vi "VLC - Play Stream&Snapshot.vi"(5 "Media Source":string="rtsp://user:password@*.*.*.*/axis-media/media.amp?videocodec=h264", 7 "Script":string, 11 "error in (no error)":errorcluster) -> (15 "error out":errorcluster)   [LabVIEW 2012]
uses:
  <vilib>/Utility/sysdir.llb/System Directory Type.ctl
  System.Windows.Forms
panel:
  in  "PictureBox":refnum<k24>(container)
  in  "Snap":bool
  # "http://www.videolan.org/developers/vlc/doc/doxygen/html/modules.html"
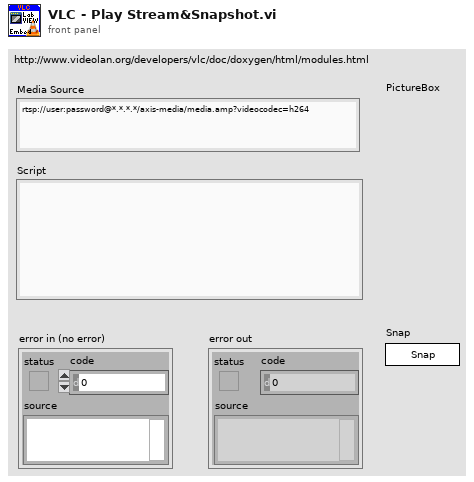
[diagram p1: front panel]
types:
  T1 = typedef "System Directory Type.ctl" = i32
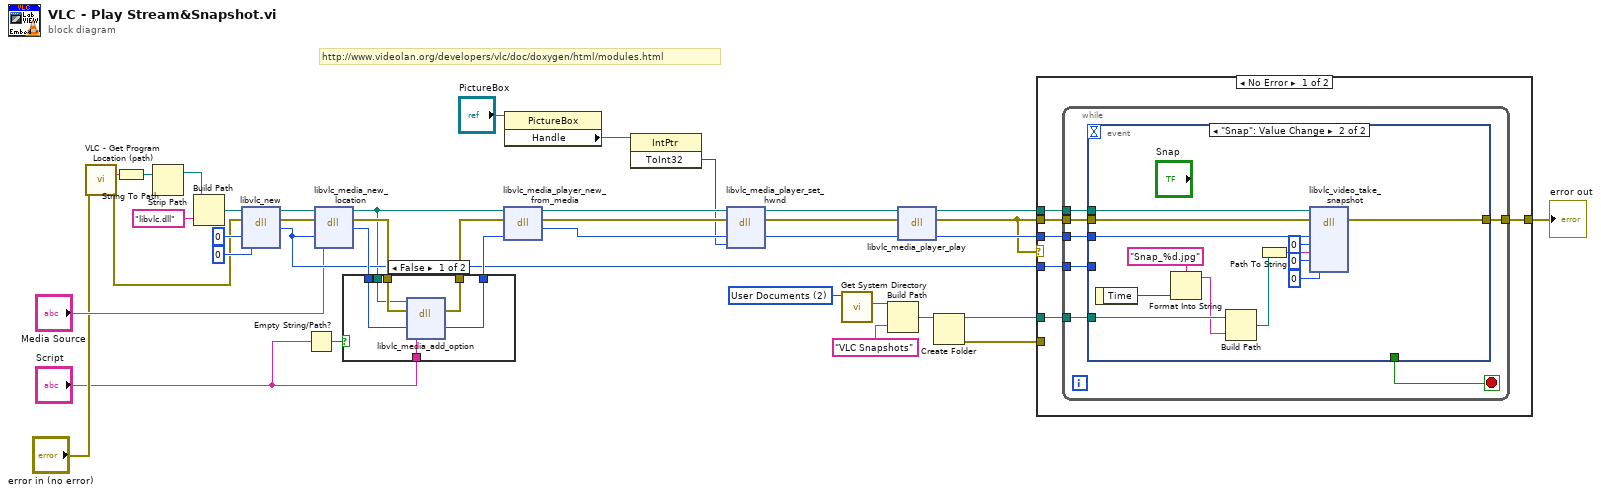
[diagram p0: block diagram]
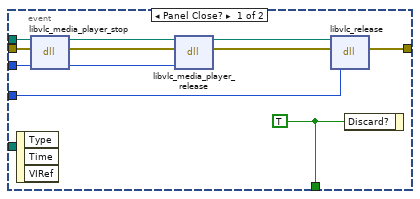
[diagram p2: hidden frame]
diagram:
  w6 = T1 2 items=["User Home"=0, "User Desktop"=1, "User Documents"=2, "User Application Data"=3, "User Preferences"=4, "User Temporary"=5, "Public Documents"=6, "Public Application Data"=7, "Public Preferences"=8, "Public Cache"=13, "System Core Libraries"=9, "System Installed Libraries"=10, "Application Files"=11, "Boot Volume Root"=12] ("system directory type")
  # "http://www.videolan.org/developers/vlc/doc/doxygen/html/modules.html"
  n1 = call "VLC - Get Program Location (path).vi"("error in (no error)"="error in (no error)") -> ("VLC path"=w22:string, "error out"=w15:errorcluster)  [unwired: 13 in]
  n2 = String To Path(string=w22) -> (path=w21:path)
  n3 = Strip Path(path=w21) -> (stripped path=w20:path)  [unwired: 1 out]
  n4 = Build Path(base path=w20, name or relative path="libvlc.dll") -> (appended path=w18:path)
  n5 = dll-call lib="C:/Program Files (x86)/VideoLAN/VLC/libvlc.dll" fn="libvlc_new"(path in=w18, error in=w15, "argc"=i16 0, "argv"=u8 0) -> (path out=w26:path, error out=w29:errorcluster, "return type"=w35:i32)  [unwired: 3 in]
  n6 = Empty String/Path?(string/path="Script") -> (empty?=w13:bool)
  n7 = dll-call lib="C:/Program Files (x86)/VideoLAN/VLC/libvlc.dll" fn="libvlc_media_new_location"(path in=w26, error in=w29, "p_instance"=w35, "path"="Media Source") -> (path out=w10:path, error out=w36:errorcluster, "return type"=w37:i32)  [unwired: 3 in]
  n8 = case shown="False" w13 {
    tunnel: w36 -> [w45 w47]
    tunnel: w37 -> [w44 w46]
    tunnel: [w43 w46] -> w38
    tunnel: [w42 w47] -> w39
    tunnel: "Script" -> [w41 _]
    tunnel: w10 -> [w40 _]
    frame False {
      n9 = dll-call lib="C:/Program Files (x86)/VideoLAN/VLC/libvlc.dll" fn="libvlc_media_add_option"(path in=w40, error in=w45, "p_md"=w44, "ppsz_options"=w41) -> (error out=w42:errorcluster, "p_md"=w43:i32)  [unwired: 3 in, 1 out]
    }
    frame True {
    }
  }
  n10 = dll-call lib="C:/Program Files (x86)/VideoLAN/VLC/libvlc.dll" fn="libvlc_media_player_new_from_media"(path in=w10, error in=w39, "p_md"=w38) -> (path out=w25:path, error out=w32:errorcluster, "return type"=w30:i32)  [unwired: 2 in]
  n11 = property class="PictureBox"(reference="PictureBox") -> ("Handle"=w8:refnum<k24>)  [unwired: 1 in, 2 out]
  n12 = invoke class="IntPtr" method="ToInt32"(reference=w8) -> ("ToInt32"=w7:i32)  [unwired: 2 in, 2 out]
  n13 = dll-call lib="C:/Program Files (x86)/VideoLAN/VLC/libvlc.dll" fn="libvlc_media_player_set_hwnd"(path in=w25, error in=w32, "p_mi"=w30, "drawable"=w7) -> (path out=w24:path, error out=w33:errorcluster, "p_mi"=w31:i32)  [unwired: 3 in]
  n14 = call <vilib>:"Get System Directory.vi"("system directory type"=w6) -> ("system directory"=w5:path)  [unwired: 10 in]
  n15 = Build Path(base path=w5, name or relative path="VLC Snapshots") -> (appended path=w3:path)
  n16 = dll-call lib="C:/Program Files (x86)/VideoLAN/VLC/libvlc.dll" fn="libvlc_media_player_play"(path in=w24, error in=w33, "p_mi"=w31) -> (path out=w23:path, error out=w11:errorcluster, "p_mi"=w34:i32)  [unwired: 2 in]
  n17 = Create Folder(path (use dialog)=w3) -> (created path=w2:path, error out=w1:errorcluster)  [unwired: 2 in, 1 out]
  n18 = case shown="No Error" w11 {
    tunnel: w35 -> [w53 _]
    tunnel: w34 -> [w52 _]
    tunnel: w11 -> [w51 w85]
    tunnel: w23 -> [w50 _]
    tunnel: [w49 w85] -> w12
    tunnel: w2 -> [w48 _]
    tunnel: w1 -> [_ _]
    frame No Error {
      n19 = while {
        tunnel: w53 -> [w60]
        tunnel: w52 -> [w59]
        tunnel: w51 -> [w58]
        tunnel: w50 -> [w57]
        tunnel: [w56] -> w49
        tunnel: w48 -> [w54]
        stop <- w55 stop-if-true
        n20 = event shown="[1] \"Snap\": Value Change" {
          selector: _ -> [_ _]
          dyn-events: _ -> [_ _]
          timeout: _ -> [_ _]
          tunnel: w58 -> [w71 w79]
          tunnel: w59 -> [w70 w77]
          tunnel: w60 -> [w66 _]
          tunnel: w57 -> [w65 w80]
          tunnel: [w62 w78] -> w56
          tunnel: [w61 _] -> w55
          tunnel: w54 -> [_ w74]
          event Panel Close? {
            w61 = TRUE ("Discard?")
            n21 = event-data() -> ()  [unwired: 1 in, 3 out]
            n22 = dll-call lib="C:/Program Files (x86)/VideoLAN/VLC/libvlc.dll" fn="libvlc_media_player_stop"(path in=w65, error in=w71, "p_mi"=w70) -> (path out=w64:path, error out=w69:errorcluster, "p_mi"=w68:i32)  [unwired: 2 in]
            n23 = dll-call lib="C:/Program Files (x86)/VideoLAN/VLC/libvlc.dll" fn="libvlc_media_player_release"(path in=w64, error in=w69, "p_mi"=w68) -> (path out=w63:path, error out=w67:errorcluster)  [unwired: 3 in]
            n24 = dll-call lib="C:/Program Files (x86)/VideoLAN/VLC/libvlc.dll" fn="libvlc_release"(path in=w63, error in=w67, "p_instnace"=w66) -> (error out=w62:errorcluster)  [unwired: 3 in, 1 out]
            n25 = event-data("Discard?"=w61) -> ()  [unwired: 1 in, 1 out]
          }
          event "Snap": Value Change {
            n26 = event-data() -> ("Time"=w76:u32)  [unwired: 1 in]
            n27 = Format Into String(format string="Snap_%d.jpg", w76) -> (resulting string=w73:string)  [unwired: 2 in, 1 out]
            n28 = Build Path(base path=w74, name or relative path=w73) -> (appended path=w72:path)
            n29 = Path To String(path=w72) -> (string=w82:string)
            n30 = dll-call lib="C:/Program Files (x86)/VideoLAN/VLC/libvlc.dll" fn="libvlc_video_take_snapshot"(path in=w80, error in=w79, "p_mi"=w77, "num"=u32 0, "psz_filepath"=w82, "i_width"=u32 0, "i_height"=u32 0) -> (error out=w78:errorcluster)  [unwired: 7 in, 1 out]
          }
        }
      }
    }
    frame Error {
    }
  }
  "error out" <- w12
